vi "CTRE_Phoenix_Pigeon2_ConfigSettings.vi"(6 "timeoutMs":i32=50, 7 "Force Write":bool, 8 "error in (no error)":errorcluster, 10 "Pigeon2 Configurables":T1, 11 "PigeonIMUDevRef 2":T2={"DeviceStatus"={"status"=FALSE, "code"=0, "source"=""}, "Device Number"=0, "Type"=352321536, "Device ID"=0, "Handle"=0, "UsageFrame"=0, "Library Path"=path ""} {"Type" items=["CAN"=352321536, "TalonSRX"=33554432]}) -> (0 "error out":errorcluster, 3 "PigeonIMUDevRef":T2={"DeviceStatus"={"status"=FALSE, "code"=0, "source"=""}, "Device Number"=0, "Type"=352321536, "Device ID"=0, "Handle"=0, "UsageFrame"=0, "Library Path"=path ""} {"Type" items=["CAN"=352321536, "TalonSRX"=33554432]})   [LabVIEW 2020]
doc: "Configures everything needed from a Pigeon2\n\n<b>Pigeon2 Configurables</b> All the configs to apply to the Pigeon2"
uses:
  <vilib>/Rock Robotics/WPI/ThirdParty/Phoenix-LabVIEW/Pigeon IMU/CTRE_PigeonIMU_DeviceRef.ctl
  <vilib>/Rock Robotics/WPI/ThirdParty/Phoenix-LabVIEW/Pigeon IMU/CTRE_PigeonIMU_ConnectionType.ctl
  <vilib>/Rock Robotics/WPI/ThirdParty/Phoenix-LabVIEW/Pigeon2/controls/CTRE_Phoenix_Pigeon2_Configurables.ctl
panel:
  # "Yaw Angle needed to reach the current orientation in degrees"
  # "Configures the mounting pose of the Pigeon2\nThis is the yaw-pitch-roll teh Pigeon2 underwent to get to its current orientation,\n referenced from the robot's point of view\nThis is only necessary if the Pigeon2 is mounted at an exotic angle near the gimbal lock point or not forward.\nIf the pigeon is relatively flat and pointed forward, this is not needed"
  # "Pitch Angle needed to reach the current orientation in degrees"
  # "Roll Angle needed to reach the current orientation in degrees"
  # "Disables the temperature compensation\nfrom the Pigeon2. It is recommended that\nthis remains false"
  # "Disables the no-motion calibration from the\nPigeon2. It is recommended that this \nremains false"
  # "Enables the compass for Pigeon2\nThis is not recommended for any indoor robotics"
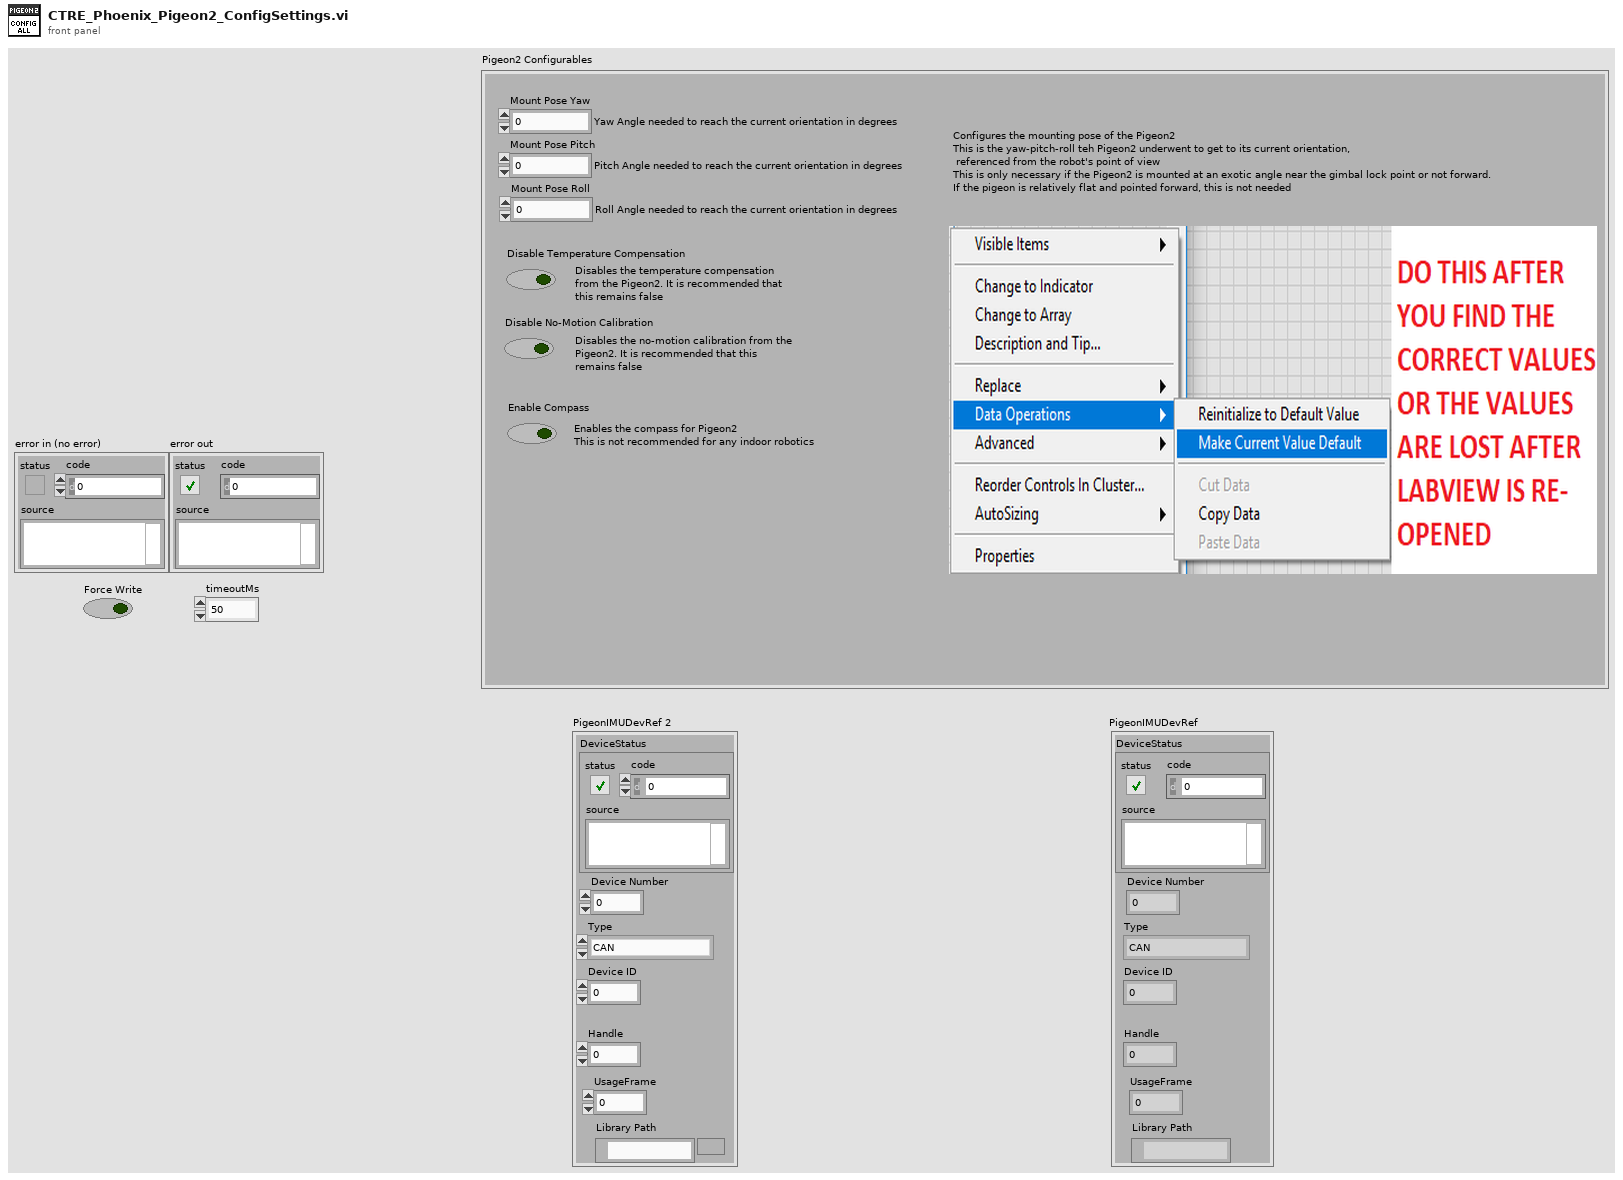
[diagram p1: front panel]
types:
  T1 = typedef "CTRE_Phoenix_Pigeon2_Configurables.ctl" = cluster{"Mount Pose Yaw":dbl, "Mount Pose Pitch":dbl, "Mount Pose Roll":dbl, "Disable Temperature Compensation":bool, "Disable No-Motion Calibration":bool, "Enable Compass":bool}
  T2 = typedef "CTRE_PigeonIMU_DeviceRef.ctl" = cluster{"DeviceStatus":errorcluster, "Device Number":u8, "Type":T3, "Device ID":u32, "Handle":u64, "UsageFrame":u32, "Library Path":path}
  T3 = typedef "CTRE_PigeonIMU_ConnectionType.ctl" = u32
  T4 = cluster{"Mount Pose Yaw":bool, "Mount Pose Pitch":bool, "Mount Pose Roll":bool, "Disable Temperature Compensation":bool, "Disable No-Motion Calibration":bool, "Enable Compass":bool}
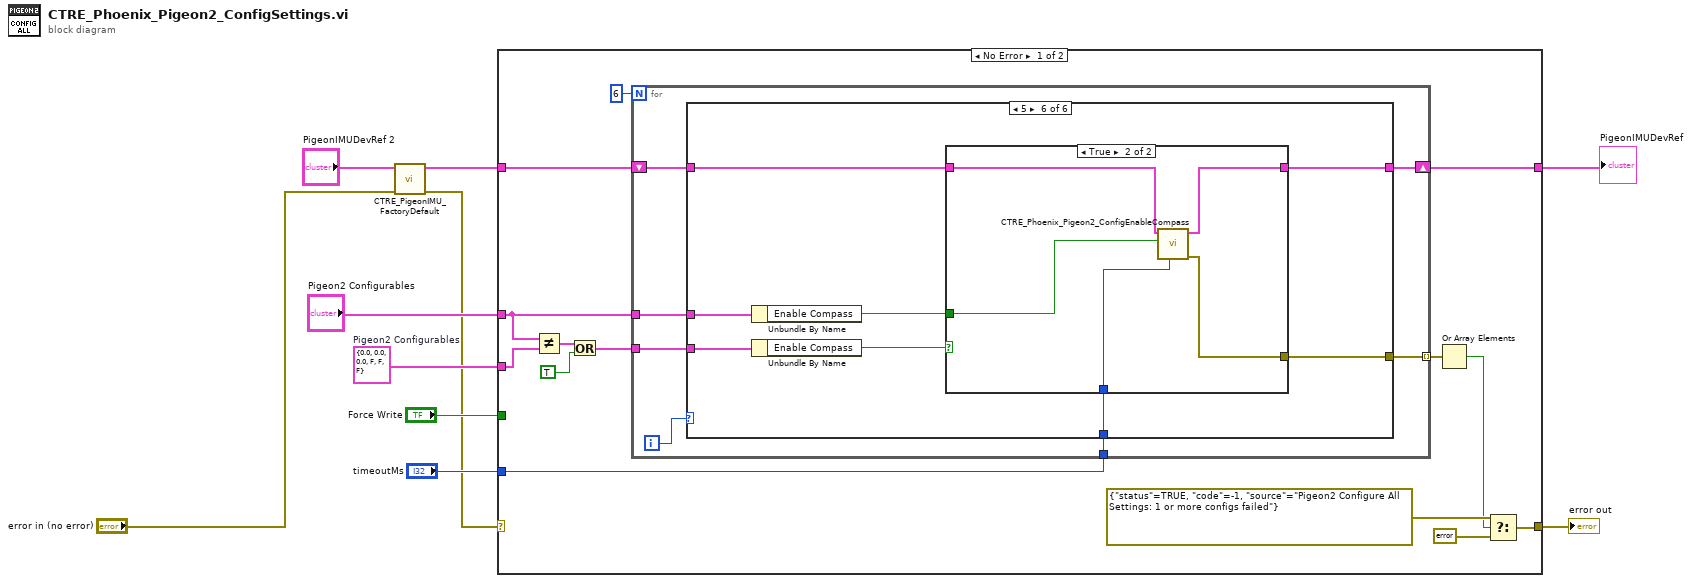
[diagram p0: block diagram]
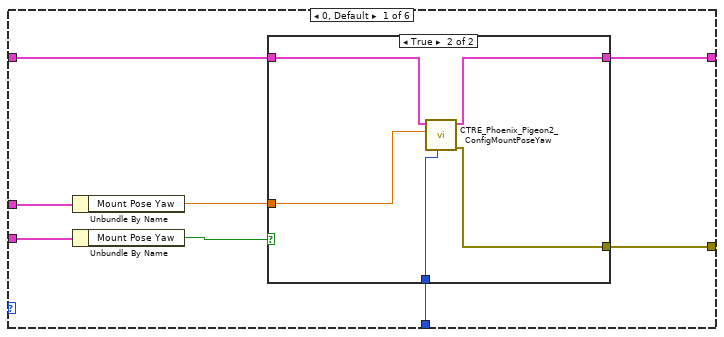
[diagram p2: hidden frame]
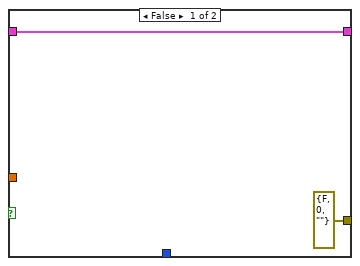
[diagram p3: hidden frame]
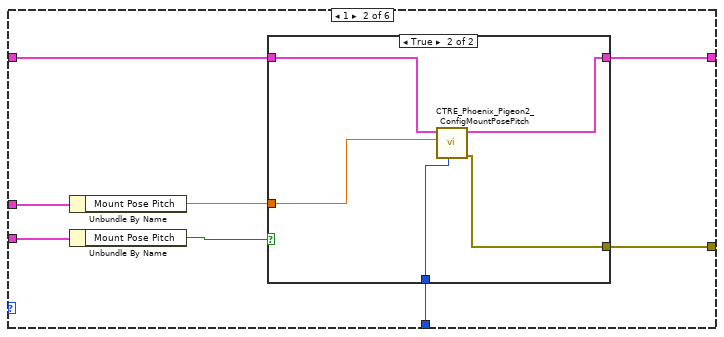
[diagram p4: hidden frame]
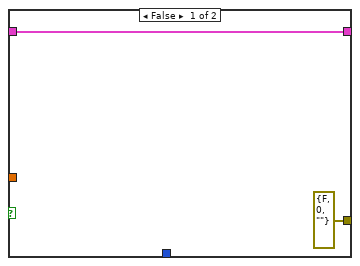
[diagram p5: hidden frame]
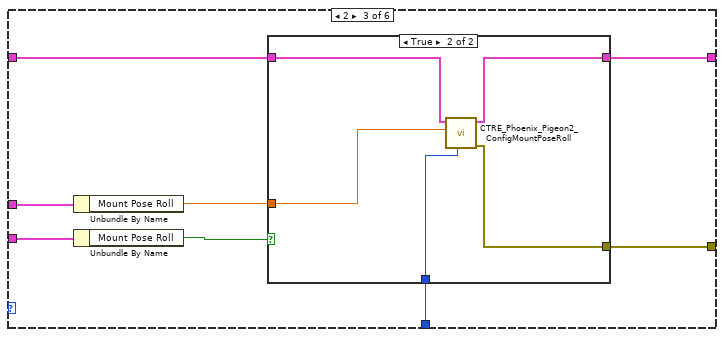
[diagram p6: hidden frame]
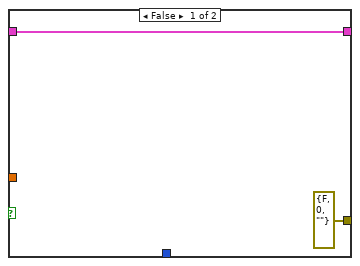
[diagram p7: hidden frame]
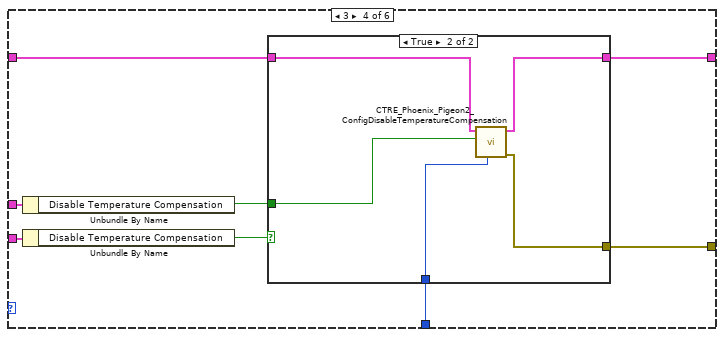
[diagram p8: hidden frame]
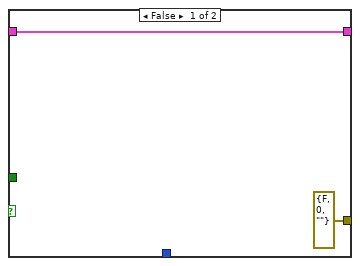
[diagram p9: hidden frame]
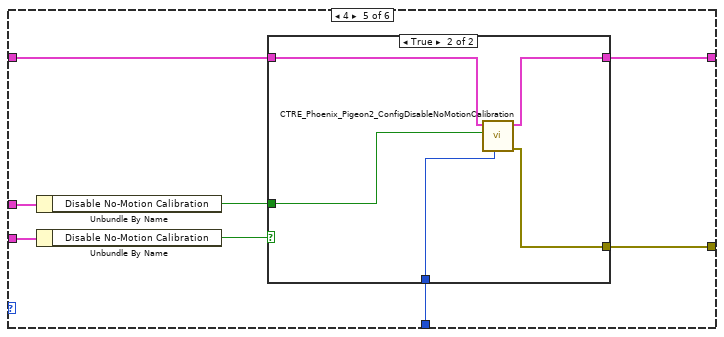
[diagram p10: hidden frame]
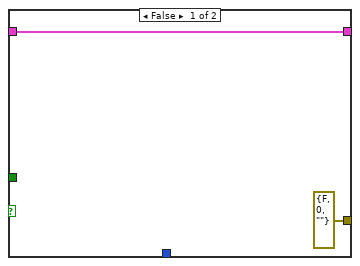
[diagram p11: hidden frame]
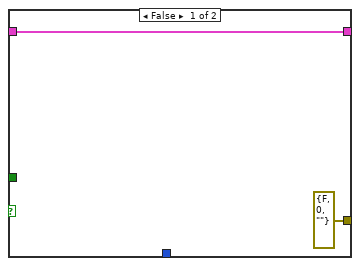
[diagram p12: hidden frame]
diagram:
  w6 = T1 {"Mount Pose Yaw"=0.0, "Mount Pose Pitch"=0.0, "Mount Pose Roll"=0.0, "Disable Temperature Compensation"=FALSE, "Disable No-Motion Calibration"=FALSE, "Enable Compass"=FALSE}  # Pigeon2 Configurables
  n1 = call <vilib>:"CTRE_PigeonIMU_FactoryDefault.vi"("error in"="error in (no error)", "PigeonIMUDevRef"="PigeonIMUDevRef 2") -> ("error out"=w1:errorcluster, "PigeonIMUDevRef"=w3:T2)  [unwired: 8 in]
  n2 = case shown="No Error" w1 {
    selector: w1 -> [_ w122]
    tunnel: w3 -> [w22 w123]
    tunnel: [w12 w123] -> w7
    tunnel: [w14 w122] -> w10
    tunnel: "timeoutMs" -> [w18 _]
    tunnel: "Force Write" -> [_ _]
    tunnel: "Pigeon2 Configurables" -> [w19 _]
    tunnel: w6 -> [w24 _]
    frame No Error {
      n3 = Not Equal?(x=w19, y=w24) -> (x != y?=w23:T4)
      n4 = Or(x=w23, y=TRUE ("Force Write")) -> (x .or. y?=w20:T4)
      n5 = for {
        N: 6 -> [_]
        shift-right: [w26] -> w12
        shift-left: w22 -> [w28]
        tunnel: w20 -> [w30]
        tunnel: w19 -> [w29]
        tunnel: w18 -> [w27]
        tunnel: [w25] -> w17 mode=indexing
        i -> [w31]
        n6 = case shown="5" w31 {
          tunnel: w30 -> [w38 w53 w68 w83 w98 w108]
          tunnel: w29 -> [w39 w54 w69 w84 w99 w109]
          tunnel: w28 -> [w35 w50 w65 w80 w95 w110]
          tunnel: w27 -> [w33 w48 w63 w78 w93 w107]
          tunnel: [w34 w49 w64 w79 w94 w111] -> w26
          tunnel: [w32 w47 w62 w77 w92 w112] -> w25
          frame 0, Default {
            n7 = Unbundle By Name(w39) -> ("Mount Pose Yaw"=w36:dbl)
            n8 = Unbundle By Name(w38) -> ("Mount Pose Yaw"=w37:bool)
            n9 = case shown="True" w37 {
              tunnel: w36 -> [_ w43]
              tunnel: w35 -> [w41 w46]
              tunnel: [w41 w45] -> w34
              tunnel: w33 -> [_ w42]
              tunnel: [errorcluster {"status"=FALSE, "code"=0, "source"=""} ("error out") w44] -> w32
              frame False {
              }
              frame True {
                n10 = call <vilib>:"CTRE_Phoenix_Pigeon2_ConfigMountPoseYaw.vi"("timeoutMs"=w42, "Yaw"=w43, "PigeonIMUDevRef"=w46) -> ("error out"=w44:errorcluster, "PigeonIMUDevRef 2"=w45:T2)  [unwired: 7 in]
              }
            }
          }
          frame 1 {
            n11 = Unbundle By Name(w54) -> ("Mount Pose Pitch"=w51:dbl)
            n12 = Unbundle By Name(w53) -> ("Mount Pose Pitch"=w52:bool)
            n13 = case shown="True" w52 {
              tunnel: w51 -> [_ w58]
              tunnel: w50 -> [w56 w61]
              tunnel: [w56 w60] -> w49
              tunnel: w48 -> [_ w57]
              tunnel: [errorcluster {"status"=FALSE, "code"=0, "source"=""} ("error out") w59] -> w47
              frame False {
              }
              frame True {
                n14 = call <vilib>:"CTRE_Phoenix_Pigeon2_ConfigMountPosePitch.vi"("timeoutMs"=w57, "Pitch"=w58, "PigeonIMUDevRef"=w61) -> ("error out"=w59:errorcluster, "PigeonIMUDevRef 2"=w60:T2)  [unwired: 7 in]
              }
            }
          }
          frame 2 {
            n15 = Unbundle By Name(w69) -> ("Mount Pose Roll"=w66:dbl)
            n16 = Unbundle By Name(w68) -> ("Mount Pose Roll"=w67:bool)
            n17 = case shown="True" w67 {
              tunnel: w66 -> [_ w74]
              tunnel: w65 -> [w71 w75]
              tunnel: [w71 w76] -> w64
              tunnel: w63 -> [_ w72]
              tunnel: [errorcluster {"status"=FALSE, "code"=0, "source"=""} ("error out") w73] -> w62
              frame False {
              }
              frame True {
                n18 = call <vilib>:"CTRE_Phoenix_Pigeon2_ConfigMountPoseRoll.vi"("timeoutMs"=w72, "Roll"=w74, "PigeonIMUDevRef"=w75) -> ("error out"=w73:errorcluster, "PigeonIMUDevRef 2"=w76:T2)  [unwired: 7 in]
              }
            }
          }
          frame 3 {
            n19 = Unbundle By Name(w84) -> ("Disable Temperature Compensation"=w81:bool)
            n20 = Unbundle By Name(w83) -> ("Disable Temperature Compensation"=w82:bool)
            n21 = case shown="True" w82 {
              tunnel: w81 -> [_ w88]
              tunnel: w80 -> [w86 w91]
              tunnel: [w86 w90] -> w79
              tunnel: w78 -> [_ w87]
              tunnel: [errorcluster {"status"=FALSE, "code"=0, "source"=""} ("error out") w89] -> w77
              frame False {
              }
              frame True {
                n22 = call <vilib>:"CTRE_Phoenix_Pigeon2_ConfigDisableTemperatureCompensation.vi"("timeoutMs"=w87, "disable"=w88, "PigeonIMUDevRef"=w91) -> ("error out"=w89:errorcluster, "PigeonIMUDevRef 2"=w90:T2)  [unwired: 7 in]
              }
            }
          }
          frame 4 {
            n23 = Unbundle By Name(w99) -> ("Disable No-Motion Calibration"=w96:bool)
            n24 = Unbundle By Name(w98) -> ("Disable No-Motion Calibration"=w97:bool)
            n25 = case shown="True" w97 {
              tunnel: w96 -> [_ w104]
              tunnel: w95 -> [w101 w103]
              tunnel: [w101 w106] -> w94
              tunnel: w93 -> [_ w102]
              tunnel: [errorcluster {"status"=FALSE, "code"=0, "source"=""} ("error out") w105] -> w92
              frame False {
              }
              frame True {
                n26 = call <vilib>:"CTRE_Phoenix_Pigeon2_ConfigDisableNoMotionCalibration.vi"("timeoutMs"=w102, "disable"=w104, "PigeonIMUDevRef"=w103) -> ("error out"=w105:errorcluster, "PigeonIMUDevRef 2"=w106:T2)  [unwired: 7 in]
              }
            }
          }
          frame 5 {
            n27 = Unbundle By Name(w109) -> ("Enable Compass"=w113:bool)
            n28 = Unbundle By Name(w108) -> ("Enable Compass"=w114:bool)
            n29 = case shown="True" w114 {
              tunnel: w113 -> [_ w117]
              tunnel: w110 -> [w116 w121]
              tunnel: [w116 w120] -> w111
              tunnel: w107 -> [_ w118]
              tunnel: [errorcluster {"status"=FALSE, "code"=0, "source"=""} ("error out") w119] -> w112
              frame False {
              }
              frame True {
                n30 = call <vilib>:"CTRE_Phoenix_Pigeon2_ConfigEnableCompass.vi"("timeoutMs"=w118, "enable"=w117, "PigeonIMUDevRef"=w121) -> ("error out"=w119:errorcluster, "PigeonIMUDevRef 2"=w120:T2)  [unwired: 7 in]
              }
            }
          }
        }
      }
      n31 = Or Array Elements(Boolean array=w17) -> (logical OR=w13:bool)
      n32 = Select(t=errorcluster {"status"=TRUE, "code"=-1, "source"="Pigeon2 Configure All Settings: 1 or more configs failed"} ("error out 2"), s=w13, f=errorcluster {"status"=FALSE, "code"=0, "source"=""} ("error out 2")) -> (s? t:f=w14:errorcluster)
    }
    frame Error {
    }
  }
  "error out" <- w10
  "PigeonIMUDevRef" <- w7
